vi "test-VAttributes-DataToVattributes(simpleTD).vi"(8 "error in (no error)":errorcluster, 11 "TestCase in":refnum<class "MyTestCase.lvclass">) -> (0 "error out":errorcluster, 3 "TestCase out":refnum<class "MyTestCase.lvclass">)   [LabVIEW 2019, in "MyTestCase.lvclass"]
uses:
  MyTestCase.lvclass
  <vilib>/addons/_JKI Toolkits/VI Tester/TestCase.llb/TestCase.lvclass
  C:/Program Files (x86)/National Instruments/LabVIEW 2019/vi.lib/addons/_JKI Toolkits/VI Tester/TestCase.llb/TestCase.lvclass
panel:
  out "data 5":variant
  out "data 3":variant
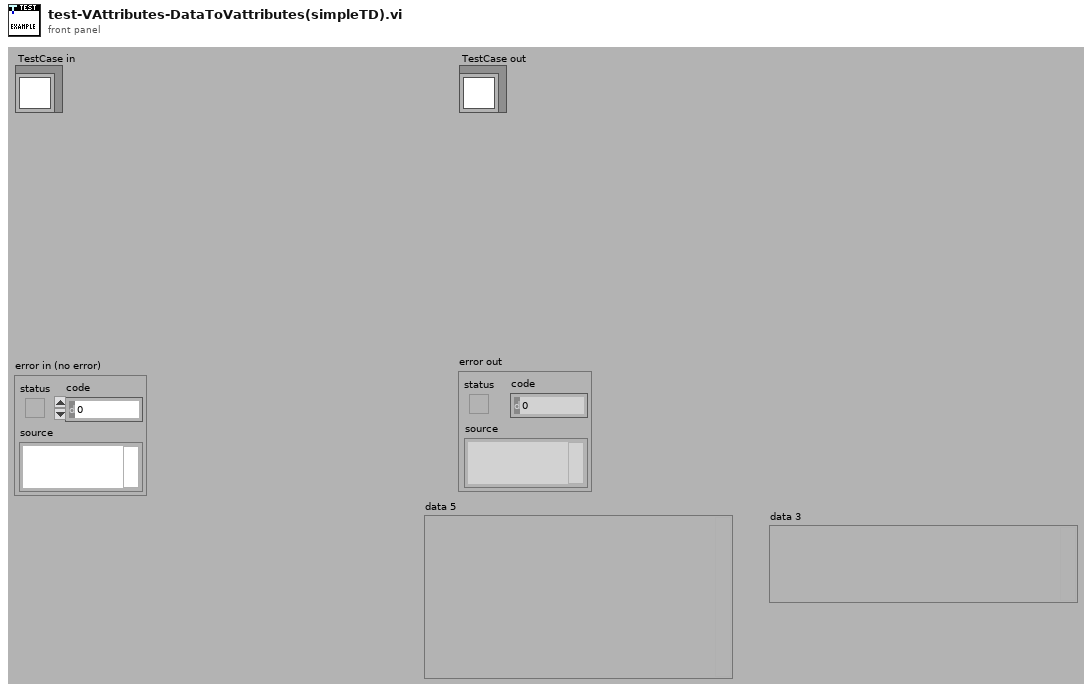
[diagram p1: front panel]
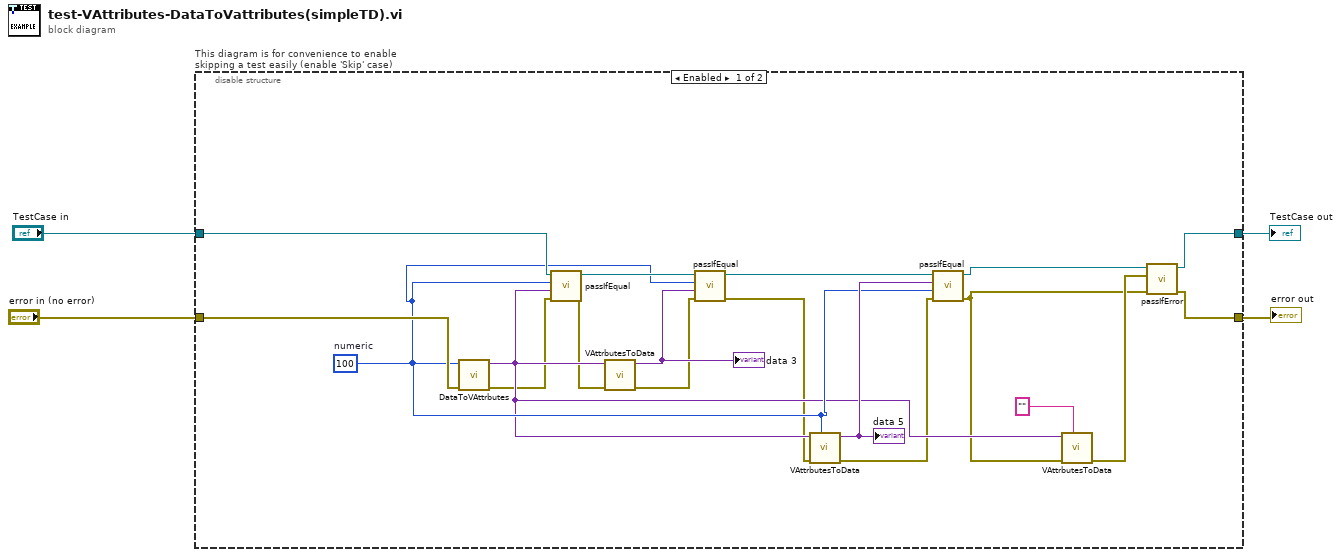
[diagram p0: block diagram]
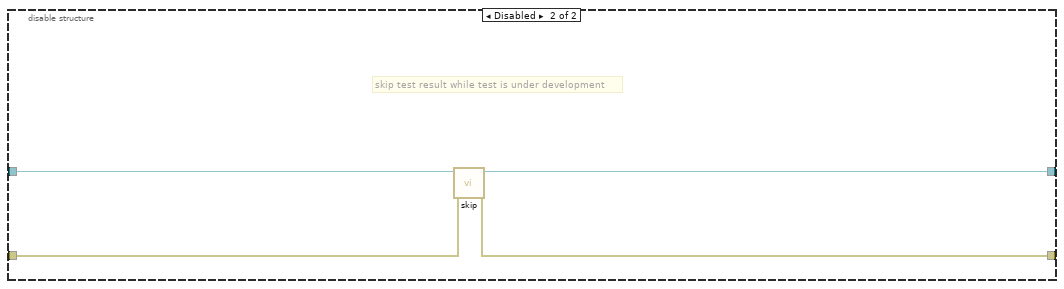
[diagram p2: hidden frame]
diagram:
  n1 = disable-structure "This diagram is for convenience to enable skipping a test easily (enable 'Skip' case)" shown="Enabled" {
    disable-tunnel: "TestCase in" -> [w22 w27]
    disable-tunnel: [w6 w25] -> w1
    disable-tunnel: [w7 w26] -> w3
    disable-tunnel: "error in (no error)" -> [w23 w24]
    frame Enabled {
      w17 = 100  # numeric
      n2 = call "DataToVAttrbutes.vi"("error in (no error)"=w23, "data"=w17) -> ("error out"=w12:errorcluster, "VAttributes"=w15:variant)  [unwired: 8 in]
      n3 = call-dynamic "passIfEqual.vi"("error in (no error)"=w12, "y"=w15, "x"=w17, "TestCase in"=w22) -> ("error out"=w11:errorcluster, "TestCase out"=w20:refnum<class "MyTestCase.lvclass">)  [unwired: 6 in]
      n4 = call "VAttrbutesToData.vi"("error in (no error)"=w11, "VAttributes"=w15) -> ("error out"=w10:errorcluster, "data"=w21:variant)  [unwired: 8 in]
      "data 3" <- w21
      n5 = call-dynamic "passIfEqual.vi"("error in (no error)"=w10, "y"=w21, "x"=w17, "TestCase in"=w20) -> ("error out"=w9:errorcluster, "TestCase out"=w19:refnum<class "MyTestCase.lvclass">)  [unwired: 6 in]
      n6 = call "VAttrbutesToData.vi"("Prototype"=w17, "error in (no error)"=w9, "VAttributes"=w15) -> ("error out"=w8:errorcluster, "data"=w18:variant)  [unwired: 7 in]
      "data 5" <- w18
      n7 = call-dynamic "passIfEqual.vi"("error in (no error)"=w8, "y"=w17, "x"=w18, "TestCase in"=w19) -> ("error out"=w5:errorcluster, "TestCase out"=w13:refnum<class "MyTestCase.lvclass">)  [unwired: 6 in]
      n8 = call "VAttrbutesToData.vi"("Prototype"="", "error in (no error)"=w5, "VAttributes"=w15) -> ("error out"=w14:errorcluster)  [unwired: 7 in, 1 out]
      n9 = call-dynamic "passIfError.vi"("error in (no error)"=w5, "error"=w14, "TestCase in"=w13) -> ("error out"=w7:errorcluster, "TestCase out"=w6:refnum<class "MyTestCase.lvclass">)  [unwired: 7 in]
    }
    frame Disabled {
      # "skip test result while test is under development"
      n10 = call <vilib>:"skip.vi"("error in (no error)"=w24, "TestCase in"=w27) -> ("error out"=w26:errorcluster, "TestCase out"=w25:refnum<class "MyTestCase.lvclass">)  [unwired: 8 in]
    }
  }
  "error out" <- w3
  "TestCase out" <- w1
